vi "cursor_add.vi"(7 "xy_graph_reference":refnum<vi>, 8 "error in (no error)":errorcluster, 11 "cursor_configuration":T1) -> (0 "error out":errorcluster)   [LabVIEW 2015, in "lv-graph.lvlib"]
doc: "This VI can be used to append or update a single cursor indexed by the active_cursor element."
uses:
  lv-graph.lvlib
  _controls/configuration_cursor.ctl
panel:
  in  "pad_name?":bool
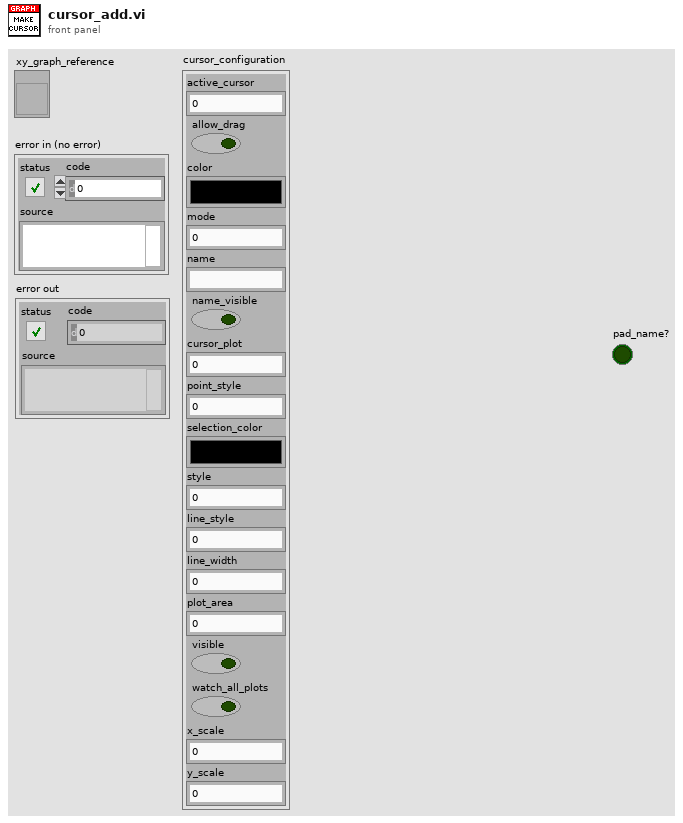
[diagram p1: front panel]
types:
  T1 = typedef "lv-graph.lvlib/configuration_cursor.ctl" = cluster{"active_cursor":u32, "allow_drag":bool, "color":u32, "mode":u32, "name":string, "name_visible":bool, "cursor_plot":i32, "point_style":u8, "selection_color":u32, "style":u8, "line_style":u8, "line_width":u8, "plot_area":i32, "visible":bool, "watch_all_plots":bool, "x_scale":u32, "y_scale":u32}
  T2 = typedef "LVCursorListTypeDef.ctl" = cluster{"Name":string, "Color":u32, "Style":u8, "Point Style":u8, "Name Visible":bool, "Allow Drag":bool, "Cursor Mode":u32, "Plot":i32, "Index":i32, "Position":cluster{"X":dbl, "Y":dbl}, "X Scale":u32, "Y Scale":u32, "Watch Plots":i32[], "Watch All Plots":bool, "Plot Area":i32, "Label Offset":cluster{"X":dbl, "Y":dbl}}[]
  T3 = cluster{"Name":string, "Color":u32, "Style":u8, "Point Style":u8, "Name Visible":bool, "Allow Drag":bool, "Cursor Mode":u32, "Plot":i32, "Index":i32, "Position":cluster{"X":dbl, "Y":dbl}, "X Scale":u32, "Y Scale":u32, "Watch Plots":i32[], "Watch All Plots":bool, "Plot Area":i32, "Label Offset":cluster{"X":dbl, "Y":dbl}}
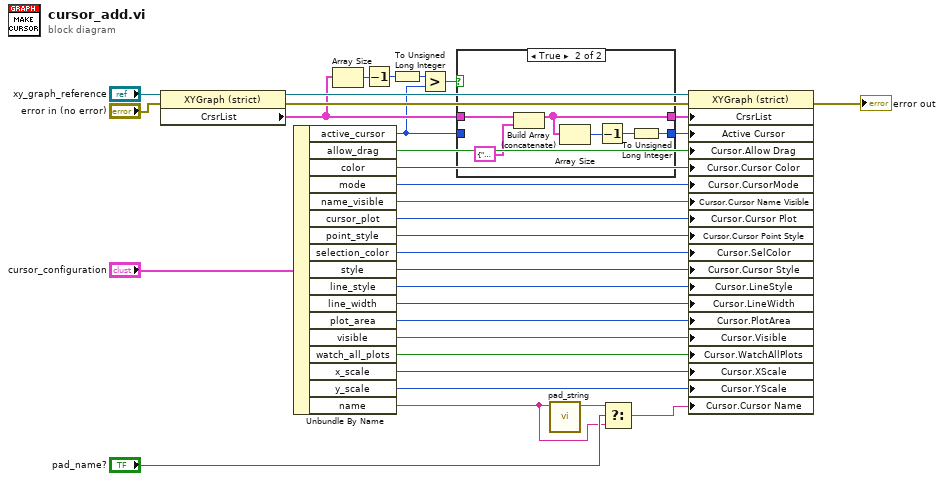
[diagram p0: block diagram]
diagram:
  n1 = property class="XYGraph (strict)"(reference="xy_graph_reference", error in="error in (no error)") -> (reference out=w11:refnum<vi>, error out=w9:errorcluster, "CrsrList"=w5:T2)
  n2 = Unbundle By Name("cursor_configuration") -> ("active_cursor"=w3:u32, "allow_drag"=w30:bool, "color"=w29:u32, "mode"=w28:u32, "name_visible"=w27:bool, "cursor_plot"=w26:i32, "point_style"=w25:u8, "selection_color"=w24:u32, "style"=w23:u8, "line_style"=w22:u8, "line_width"=w21:u8, "plot_area"=w20:i32, "visible"=w19:bool, "watch_all_plots"=w18:bool, "x_scale"=w17:u32, "y_scale"=w16:u32, "name"=w15:string)
  n3 = Array Size(array=w5) -> (size(s)=w8:i32)
  n4 = Decrement(x=w8) -> (x-1=w7:i32)
  n5 = To Unsigned Long Integer(number=w7) -> (unsigned 32bit integer=w1:u32)
  n6 = Greater?(x=w1, y=w3) -> (0:w6:bool)
  n7 = case shown="True" w6 {
    tunnel: w5 -> [w35 w41]
    tunnel: [w35 w39] -> w4
    tunnel: w3 -> [w34 _]
    tunnel: [w34 w36] -> w2
    frame False {
    }
    frame True {
      n8 = Build Array (concatenate)(w41, T3 {"Name"="", "Color"=0, "Style"=0, "Point Style"=0, "Name Visible"=FALSE, "Allow Drag"=FALSE, "Cursor Mode"=0, "Plot"=0, "Index"=0, "Position"={"X"=0.0, "Y"=0.0}, "X Scale"=0, "Y Scale"=0, "Watch Plots"=[], "Watch All Plots"=FALSE, "Plot Area"=0, "Label Offset"={"X"=0.0, "Y"=0.0}}) -> (w39:T2)
      n9 = Array Size(array=w39) -> (size(s)=w38:i32)
      n10 = Decrement(x=w38) -> (x-1=w37:i32)
      n11 = To Unsigned Long Integer(number=w37) -> (unsigned 32bit integer=w36:u32)
    }
  }
  n12 = call "pad_string.vi"("string"=w15) -> ("padded_string"=w14:string)  [unwired: 10 in]
  n13 = Select(t=w14, s="pad_name?", f=w15) -> (s? t:f=w13:string)
  n14 = property class="XYGraph (strict)"(reference=w11, error in=w9, "CrsrList"=w4, "Active Cursor"=w2, "Cursor.Allow Drag"=w30, "Cursor.Cursor Color"=w29, "Cursor.CursorMode"=w28, "Cursor.Cursor Name Visible"=w27, "Cursor.Cursor Plot"=w26, "Cursor.Cursor Point Style"=w25, "Cursor.SelColor"=w24, "Cursor.Cursor Style"=w23, "Cursor.LineStyle"=w22, "Cursor.LineWidth"=w21, "Cursor.PlotArea"=w20, "Cursor.Visible"=w19, "Cursor.WatchAllPlots"=w18, "Cursor.XScale"=w17, "Cursor.YScale"=w16, "Cursor.Cursor Name"=w13) -> (error out=→"error out":errorcluster)  [unwired: 1 out]
